vi "Current Max Read.vi"   [LabVIEW 2023, in "Power Supply.lvclass"]
uses:
  Power Supply.lvclass
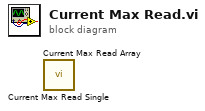
[diagram p0: block diagram]
diagram:
  n1 = call "Current Max Read Single.vi"() -> ()  [unwired: 8 in, 4 out]
  n2 = call "Current Max Read Array.vi"() -> ()  [unwired: 8 in, 4 out]
